vi "VisualizeAnalysis.vi"() -> ()   [LabVIEW 2014, in "Visualization.lvlib" / "VisualizeAnalysis.lvclass"]
uses:
  VisualizeAnalysis.lvclass
  VisualizeBase/VisualizeBase_class/Requests/clUserEventType.ctl
  <vilib>/event_ctls.llb/usereventprio.ctl
  <vilib>/Utility/file.llb/Read From Spreadsheet File (DBL).vi
  <vilib>/Utility/error.llb/Error Cluster From Error Code.vi
  <vilib>/ErrorRing/Error Ring.xnode
  VisualizeBase/VisualizeBase_class/VisualizeBase.lvclass
  <userlib>/NIST/NISTErrorLib/NISTErrorLib.lvlib
  Analysis/AnalysisModule/AnalysisModule.lvlib
panel:
  in  "Pause":bool
  out "Data from file":dbl[][](array[numeric])
  in  "btnOpen":bool
  out "RFE":dbl(graph)
  out "FE":dbl(graph)
  out "Data real time":dbl[](array[numeric])
  out "TVE":dbl[][](graph)
  in  "QueName":string="AnalVisQue"
  out "ErrorArray":errorcluster[](array[cluster])
  in  "btnStop":bool
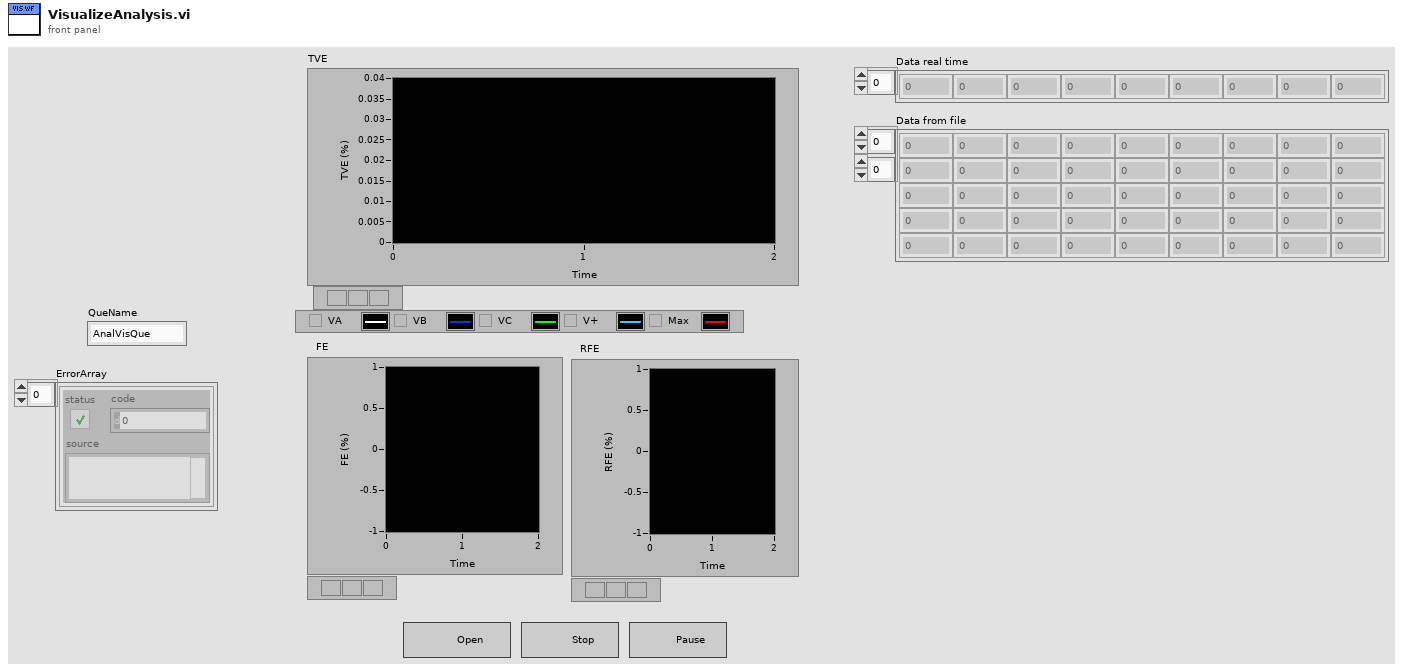
[diagram p1: front panel]
types:
  T1 = typedef "Visualization.lvlib/VisualizeBase.lvclass/clRequestEvents.ctl" = cluster{"StopRequest":refnum<user-event>, "ResetRequest":refnum<user-event>}
  T2 = typedef "AnalysisModule.lvlib/clBroadcastEvents.ctl" = cluster{"DidInit":refnum<user-event>, "StatusUpdate":refnum<user-event>, "ErrorReport":refnum<user-event>, "DidStop":refnum<user-event>, "PathToINI":refnum<user-event>, "Config":refnum<user-event>, "ResultReport":refnum<user-event>}
  T3 = typedef "Visualization.lvlib/VisualizeBase.lvclass/clUserEventType.ctl" = cluster{"BusIndex":i8, "Data":variant}
  T4 = typedef "usereventprio.ctl" = enum32{"high priority", "normal priority"}
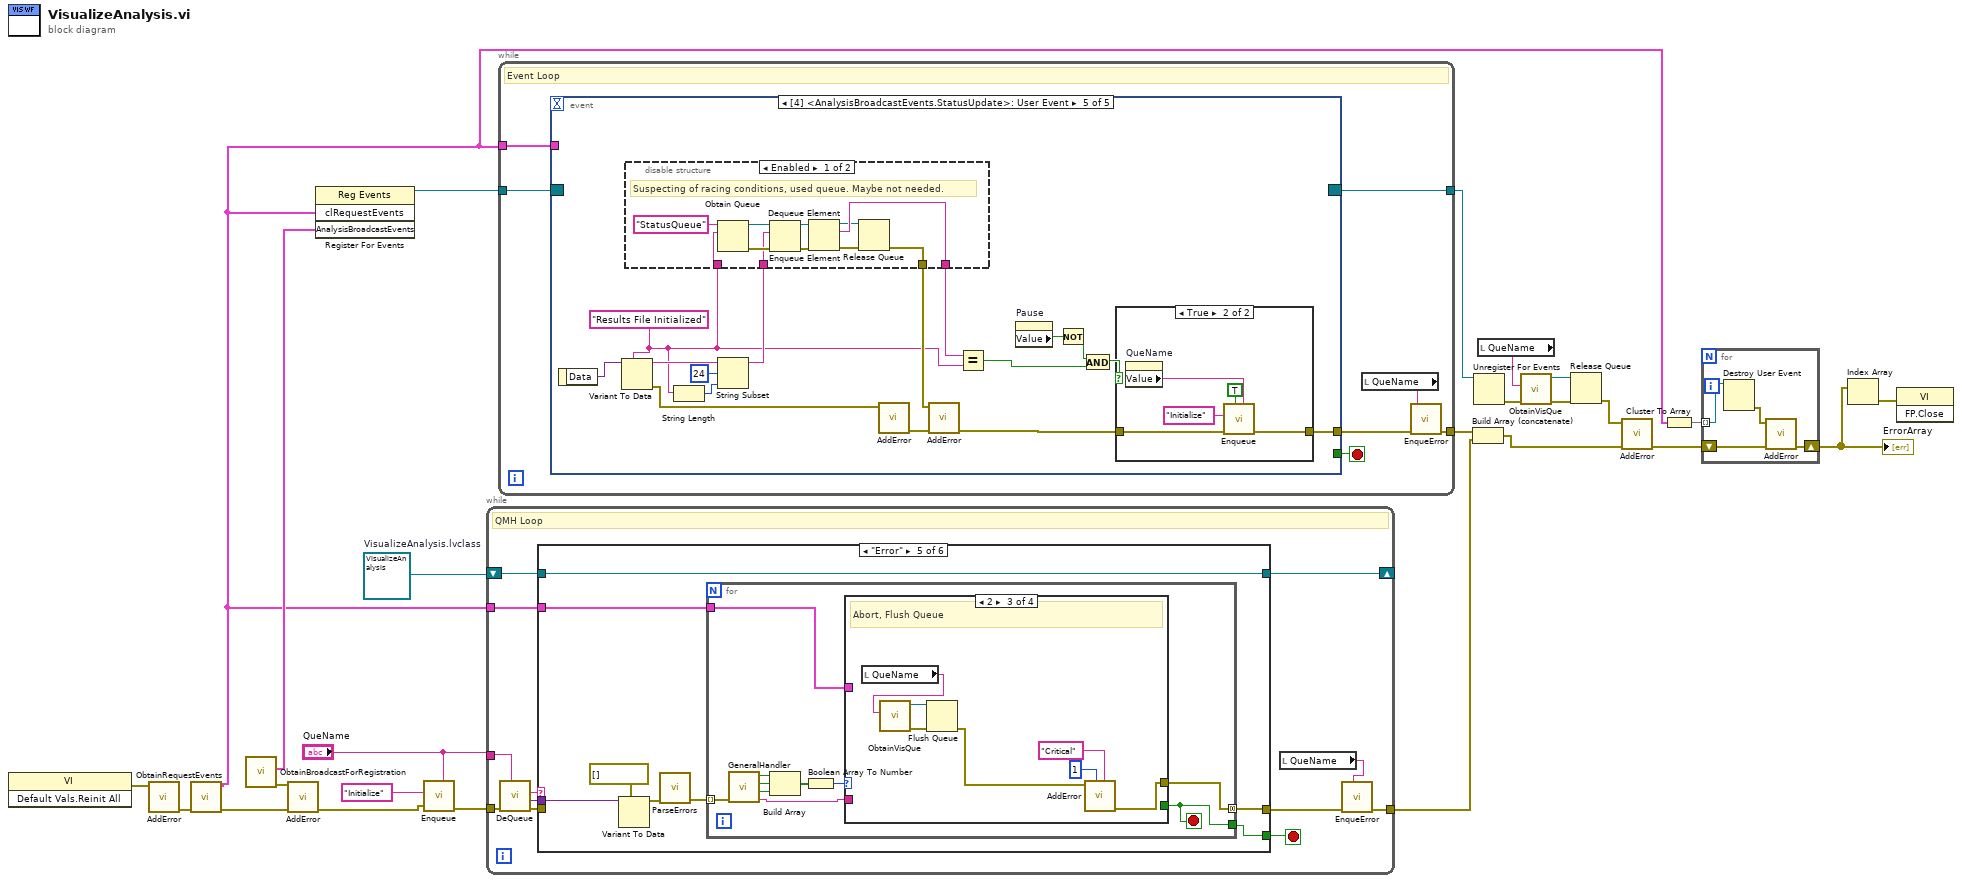
[diagram p0: block diagram]
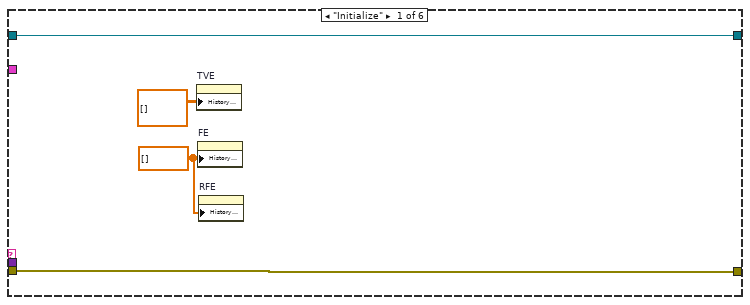
[diagram p2: hidden frame]
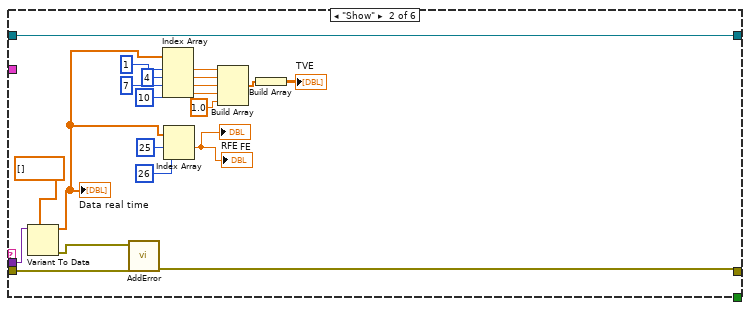
[diagram p3: hidden frame]
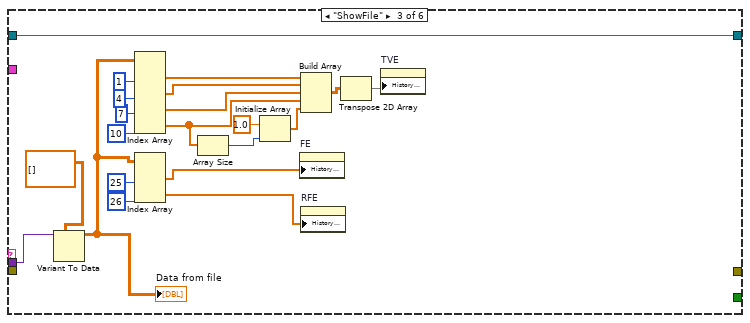
[diagram p4: hidden frame]
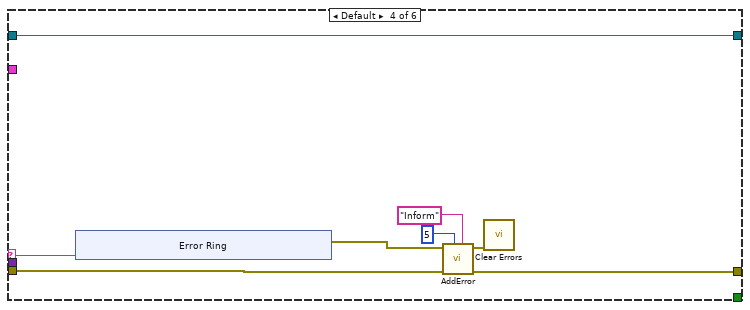
[diagram p5: hidden frame]
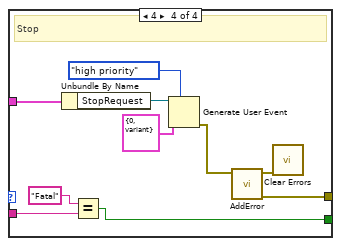
[diagram p8: hidden frame]
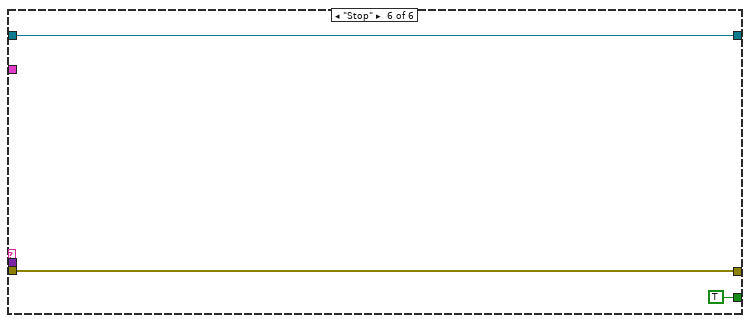
[diagram p9: hidden frame]
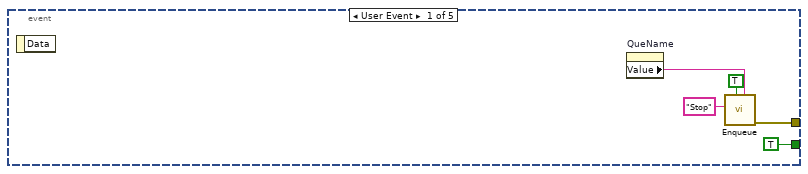
[diagram p10: hidden frame]
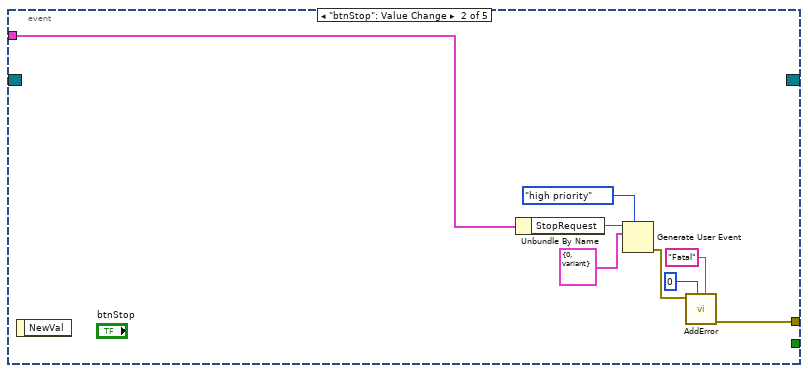
[diagram p11: hidden frame]
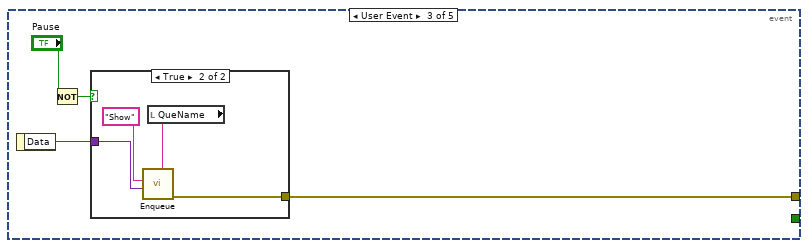
[diagram p12: hidden frame]
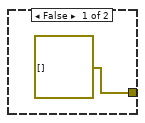
[diagram p13: hidden frame]
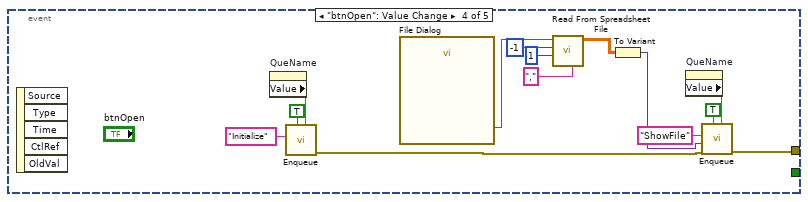
[diagram p14: hidden frame]
diagram:
  w14 = refnum<class "VisualizeAnalysis.lvclass"> refnum  # VisualizeAnalysis.lvclass
  n1 = invoke class="VI" method="Default Vals.Reinit All"() -> (error out=w21:errorcluster)  [unwired: 3 in, 2 out]
  n2 = call <userlib>:"AddError.vi"("error in (no error)"=w21) -> ("ErrorArray"=w20:errorcluster[])  [unwired: 9 in, 1 out]
  n3 = call "ObtainRequestEvents.vi"("Error"=w20) -> ("Error"=w18:errorcluster[], "clRequestEvents"=w1:T1)  [unwired: 9 in]
  n4 = call "ObtainBroadcastForRegistration.vi"() -> ("error out"=w16:errorcluster, "AnalysisBroadcastEvents"=w19:T2)  [unwired: 10 in]
  n5 = call <userlib>:"AddError.vi"("ErrorArray"=w18, "error in (no error)"=w16) -> ("ErrorArray"=w17:errorcluster[])  [unwired: 8 in, 1 out]
  n6 = register-events(w1, w19) -> (reference out=w13:refnum<event-registration>)  [unwired: 2 in, 1 out]
  n7 = call "Enqueue.vi"("QueName"="QueName", "Error"=w17, "Message"="Initialize") -> ("Error"=w24:errorcluster[])  [unwired: 8 in]
  n8 = while {
    tunnel: w24 -> [w37]
    tunnel: [w31] -> w23
    tunnel: "QueName" -> [w29]
    shift-right: [w28] -> _
    shift-left: w14 -> [w27]
    tunnel: w1 -> [w26]
    stop <- w32 stop-if-true
    # "QMH Loop"
    n9 = call "DeQueue.vi"("QueName"=w29, "Error"=w37) -> ("Error"=w34:errorcluster[], "Data"=w35:variant, "Message"=w36:string)  [unwired: 7 in]
    n10 = case shown="\"Error\"" w36 {
      selector: w36 -> [_ _ _ w91 _ _]
      tunnel: w35 -> [_ w61 w83 _ w106 _]
      tunnel: w34 -> [w41 w44 _ w89 _ w135]
      tunnel: [w41 w42 _ w88 w102 w135] -> w33
      tunnel: [_ _ _ _ w101 TRUE] -> w32
      tunnel: w27 -> [w40 w62 w81 w84 w100 w134]
      tunnel: [w40 w62 w81 w84 w100 w134] -> w28
      tunnel: w26 -> [_ _ _ _ w99 _]
      frame "Initialize" {
        w38 = dbl[] [] ("History Data")
        n11 = property on="TVE" class="WFChart (strict)"("History Data"=dbl[][] []) -> ()  [unwired: 2 in, 2 out]
        n12 = property on="FE" class="WFChart (strict)"("History Data"=w38) -> ()  [unwired: 2 in, 2 out]
        n13 = property on="RFE" class="WFChart (strict)"("History Data"=w38) -> ()  [unwired: 2 in, 2 out]
      }
      frame "Show" {
        n14 = Variant To Data(type=dbl[] [], Variant=w61) -> (data=w49:dbl[], error out=w43:errorcluster)  [unwired: 1 in]
        "Data real time" <- w49
        n15 = call <userlib>:"AddError.vi"("ErrorArray"=w44, "error in (no error)"=w43) -> ("ErrorArray"=w42:errorcluster[])  [unwired: 8 in, 1 out]
        n16 = Index Array(array=w49, index #1=1 ("index"), index #2=4 ("index"), index #3=7 ("index"), index #4=10 ("index")) -> (element #1=w58:dbl, element #2=w53:dbl, element #3=w52:dbl, element #4=w45:dbl)
        n17 = Index Array(array=w49, index #1=25 ("index"), index #2=26 ("index")) -> (element #1=→"FE" →"RFE":dbl)  [unwired: 1 out]
        n18 = Build Array(w58, w53, w52, w45, 1.0 ("element")) -> (w57:dbl[])
        n19 = Build Array(w57) -> (→"TVE":dbl[][])
      }
      frame "ShowFile" {
        n20 = Variant To Data(type=dbl[][] [], Variant=w83) -> (data=w71:dbl[][])  [unwired: 1 in, 1 out]
        "Data from file" <- w71
        n21 = Index Array(array=w71, index (col) #1=1 ("disabled index (col)"), index (col) #2=4 ("index (col)"), index (col) #3=7 ("index (col)"), index (col) #4=10 ("index (col)")) -> (element #1=w76:dbl[], element #2=w75:dbl[], element #3=w74:dbl[], element #4=w66:dbl[])  [unwired: 4 in]
        n22 = Index Array(array=w71, index (col) #1=25 ("disabled index (col)"), index (col) #2=26 ("index (col)")) -> (element #1=w68:dbl[], element #2=w67:dbl[])  [unwired: 2 in]
        n23 = Array Size(array=w66) -> (size(s)=w65:i32)
        n24 = Initialize Array(1.0 ("element"), w65) -> (w63:dbl[])
        n25 = property on="FE" class="WFChart (strict)"("History Data"=w68) -> ()  [unwired: 2 in, 2 out]
        n26 = Build Array(w76, w75, w74, w66, w63) -> (w73:dbl[][])
        n27 = property on="RFE" class="WFChart (strict)"("History Data"=w67) -> ()  [unwired: 2 in, 2 out]
        n28 = Transpose 2D Array(2D array=w73) -> (transposed array=w72:dbl[][])
        n29 = property on="TVE" class="WFChart (strict)"("History Data"=w72) -> ()  [unwired: 2 in, 2 out]
      }
      frame Default {
        n30 = xnode "Error Ring"("parameter 0"=w91) -> ("error out"=w90:errorcluster)
        n31 = call <userlib>:"AddError.vi"("Severity"="Inform" ("String"), "Priority"=u8 5, "ErrorArray"=w89, "error in (no error)"=w90) -> ("ErrorArray"=w88:errorcluster[], "error out"=w87:errorcluster)  [unwired: 6 in]
        n32 = call <vilib>:"Clear Errors.vi"("error in (no error)"=w87) -> ()  [unwired: 5 in, 2 out]
      }
      frame "Error" {
        n33 = Variant To Data(type=errorcluster[] [], Variant=w106) -> (data=w104:errorcluster[])  [unwired: 1 in, 1 out]
        n34 = call <userlib>:"ParseErrors.vi"("ErrorArray"=w104) -> ("ErrorArray"=w103:errorcluster[])  [unwired: 8 in, 2 out]
        n35 = for {
          tunnel: w103 -> [w116] mode=indexing
          tunnel: [w110] -> w102 mode=concatenating
          tunnel: [w108] -> w101
          tunnel: w99 -> [w107]
          stop <- w108 stop-if-true
          n36 = call <userlib>:"GeneralHandler.vi"("error in (no error)"=w116) -> ("Severity"=w109:string, "Stop"=w113:bool, "Abort"=w114:bool, "Continue"=w115:bool)  [unwired: 7 in]
          n37 = Build Array(w115, w114, w113) -> (w112:bool[])
          n38 = Boolean Array To Number(Boolean array=w112) -> (number=w111:u32)
          n39 = case shown="2" w111 {
            tunnel: [_ _ w121 w132] -> w110
            tunnel: w109 -> [_ _ _ w127]
            tunnel: [_ _ _ w125] -> w108
            tunnel: w107 -> [_ _ _ w124]
            frame 0, Default {
              # "No Dialog"
            }
            frame 1 {
              # "Continue"
            }
            frame 2 {
              # "Abort, Flush Queue"
              n40 = local read "QueName"() -> (w117:string)
              n41 = call "ObtainVisQue.vi"("QueName"=w117) -> ("error out"=w123:errorcluster, "queue out"=w122:refnum<queue>)  [unwired: 9 in]
              n42 = Flush Queue(queue=w122, error in (no error)=w123) -> (error out=w120:errorcluster)  [unwired: 2 out]
              n43 = call <userlib>:"AddError.vi"("Severity"="Critical" ("String"), "Priority"=u8 1, "error in (no error)"=w120) -> ("ErrorArray"=w121:errorcluster[])  [unwired: 7 in, 1 out]
            }
            frame 4 {
              # "Stop"
              n44 = Unbundle By Name(w124) -> ("StopRequest"=w133:refnum<user-event>)
              n45 = Equal?(x="Fatal", y=w127) -> (x = y?=w125:bool)
              n46 = Generate User Event(priority (normal)=usereventprio."high priority", user event=w133, event data cluster=T3 {"BusIndex"=0, "Data"=variant} ("event data")) -> (error out=w131:errorcluster)  [unwired: 1 in, 1 out]
              n47 = call <userlib>:"AddError.vi"("error in (no error)"=w131) -> ("ErrorArray"=w132:errorcluster[], "error out"=w128:errorcluster)  [unwired: 9 in]
              n48 = call <vilib>:"Clear Errors.vi"("error in (no error)"=w128) -> ()  [unwired: 5 in, 2 out]
            }
          }
        }
      }
      frame "Stop" {
      }
    }
    n49 = local read "QueName"() -> (w30:string)
    n50 = call "EnqueError.vi"("QueName"=w30, "Error"=w33) -> ("Error"=w31:errorcluster[])  [unwired: 9 in]
  }
  n51 = while {
    tunnel: [w141] -> w22
    tunnel: w13 -> [w139]
    tunnel: [w138] -> w7
    tunnel: w1 -> [w137]
    stop <- w143 stop-if-true
    # "Event Loop"
    n52 = event shown="[4] <AnalysisBroadcastEvents.StatusUpdate>: User Event" {
      selector: w139 -> [_ _ _ _ _]
      dyn-events: [_ _ _ _ _] -> w138
      timeout: _ -> [_ _ _ _ _]
      tunnel: [TRUE _ _ _ _] -> w143
      tunnel: [w147 w154 w159 w174 w194] -> w142
      tunnel: w137 -> [_ w149 _ _ _]
      event User Event {
        n53 = event-data() -> ()  [unwired: 1 in, 1 out]
        n54 = property on="QueName" class="Str"() -> ("Value"=w144:string)  [unwired: 2 in, 2 out]
        n55 = call "Enqueue.vi"("QueName"=w144, "Priority? (F)"=TRUE, "Message"="Stop") -> ("Error"=w147:errorcluster[])  [unwired: 8 in]
      }
      event "btnStop": Value Change {
        n56 = event-data() -> ()  [unwired: 1 in, 1 out]
        n57 = Unbundle By Name(w149) -> ("StopRequest"=w155:refnum<user-event>)
        n58 = Generate User Event(priority (normal)=usereventprio."high priority", user event=w155, event data cluster=T3 {"BusIndex"=0, "Data"=variant} ("event data")) -> (error out=w156:errorcluster)  [unwired: 1 in, 1 out]
        n59 = call <userlib>:"AddError.vi"("Severity"="Fatal" ("String"), "Priority"=u8 0, "error in (no error)"=w156) -> ("ErrorArray"=w154:errorcluster[])  [unwired: 7 in, 1 out]
      }
      event User Event {
        n60 = event-data() -> ("Data"=w160:variant)  [unwired: 1 in]
        n61 = Not(x="Pause") -> (.not. x?=w157:bool)
        n62 = case shown="True" w157 {
          tunnel: w160 -> [_ w164]
          tunnel: [errorcluster[] [] ("Error") w163] -> w159
          frame False {
          }
          frame True {
            n63 = local read "QueName"() -> (w165:string)
            n64 = call "Enqueue.vi"("QueName"=w165, "Data"=w164, "Message"="Show") -> ("Error"=w163:errorcluster[])  [unwired: 8 in]
          }
        }
      }
      event "btnOpen": Value Change {
        n65 = event-data() -> ()  [unwired: 1 in, 5 out]
        n66 = property on="QueName" class="Str"() -> ("Value"=w171:string)  [unwired: 2 in, 2 out]
        n67 = call "Enqueue.vi"("QueName"=w171, "Priority? (F)"=TRUE, "Message"="Initialize") -> ("Error"=w168:errorcluster[])  [unwired: 8 in]
        n68 = call "File Dialog"() -> ("selected path"=w179:path)  [unwired: 12 in, 3 out]
        n69 = call-poly <vilib>:"Read From Spreadsheet File.vi"("delimiter (\\t)"="," ("delimiter (\\t)"), "start of read offset (chars.:0)"=1, "number of rows (all:-1)"=-1, "file path (dialog if empty)"=w179) -> ("all rows"=w173:dbl[][])  [unwired: 3 in, 4 out]
        n70 = To Variant(anything=w173) -> (Variant=w172:variant)
        n71 = property on="QueName" class="Str"() -> ("Value"=w175:string)  [unwired: 2 in, 2 out]
        n72 = call "Enqueue.vi"("QueName"=w175, "Priority? (F)"=TRUE, "Error"=w168, "Data"=w172, "Message"="ShowFile") -> ("Error"=w174:errorcluster[])  [unwired: 6 in]
      }
      event User Event {
        w184 = "Results File Initialized" ("Status")
        n73 = event-data() -> ("Data"=w195:variant)  [unwired: 1 in]
        n74 = Variant To Data(type=w184, Variant=w195) -> (data=w192:string, error out=w189:errorcluster)  [unwired: 1 in]
        n75 = String Length(string=w184) -> (length=w185:i32)
        n76 = String Subset(string=w192, offset (0)=24, length (rest)=w185) -> (substring=w187:string)
        n77 = disable-structure shown="Enabled" {
          disable-tunnel: [w199 w207] -> w191
          disable-tunnel: [w196 _] -> w188
          disable-tunnel: w187 -> [w201 w207]
          disable-tunnel: w184 -> [w200 _]
          frame Enabled {
            # "Suspecting of racing conditions, used queue. Maybe not needed."
            n78 = Obtain Queue(name (unnamed)="StatusQueue", element data type=w200) -> (queue out=w205:refnum<queue>, error out=w203:errorcluster)  [unwired: 3 in, 1 out]
            n79 = Enqueue Element(queue=w205, element=w201, error in (no error)=w203) -> (queue out=w204:refnum<queue>, error out=w202:errorcluster)  [unwired: 1 in, 1 out]
            n80 = Dequeue Element(queue=w204, error in (no error)=w202) -> (queue out=w198:refnum<queue>, element=w199:string, error out=w197:errorcluster)  [unwired: 1 in, 1 out]
            n81 = Release Queue(queue=w198, error in (no error)=w197) -> (error out=w196:errorcluster)  [unwired: 1 in, 2 out]
          }
          frame Disabled {
          }
        }
        n82 = call <userlib>:"AddError.vi"("error in (no error)"=w189) -> ("ErrorArray"=w190:errorcluster[])  [unwired: 9 in, 1 out]
        n83 = call <userlib>:"AddError.vi"("ErrorArray"=w190, "error in (no error)"=w188) -> ("ErrorArray"=w193:errorcluster[])  [unwired: 8 in, 1 out]
        n84 = Equal?(x=w191, y=w184) -> (x = y?=w182:bool)
        n85 = property on="Pause" class="Bool (strict)"() -> ("Value"=w181:bool)  [unwired: 2 in, 2 out]
        n86 = Not(x=w181) -> (.not. x?=w180:bool)
        n87 = And(x=w180, y=w182) -> (x .and. y?=w183:bool)
        n88 = case shown="True" w183 {
          tunnel: [w208 w210] -> w194
          tunnel: w193 -> [w208 w209]
          frame False {
          }
          frame True {
            n89 = property on="QueName" class="Str"() -> ("Value"=w211:string)  [unwired: 2 in, 2 out]
            n90 = call "Enqueue.vi"("QueName"=w211, "Priority? (F)"=TRUE, "Error"=w209, "Message"="Initialize") -> ("Error"=w210:errorcluster[])  [unwired: 7 in]
          }
        }
      }
    }
    n91 = local read "QueName"() -> (w140:string)
    n92 = call "EnqueError.vi"("QueName"=w140, "Error"=w142) -> ("Error"=w141:errorcluster[])  [unwired: 9 in]
  }
  n93 = Build Array (concatenate)(w22, w23) -> (w6:errorcluster[])
  n94 = Unregister For Events(event registration refnum=w7) -> (error out=w9:errorcluster)  [unwired: 1 in]
  n95 = local read "QueName"() -> (w3:string)
  n96 = call "ObtainVisQue.vi"("error in (no error)"=w9, "QueName"=w3) -> ("error out"=w10:errorcluster, "queue out"=w11:refnum<queue>)  [unwired: 8 in]
  n97 = Release Queue(queue=w11, error in (no error)=w10) -> (error out=w12:errorcluster)  [unwired: 1 in, 2 out]
  n98 = call <userlib>:"AddError.vi"("ErrorArray"=w6, "error in (no error)"=w12) -> ("ErrorArray"=w2:errorcluster[])  [unwired: 8 in, 1 out]
  n99 = Cluster To Array(cluster=w1) -> (array=w8:refnum<user-event>[])
  n100 = for {
    tunnel: w8 -> [w217] mode=indexing
    shift-right: [w216] -> w5
    shift-left: w2 -> [w215]
    n101 = Destroy User Event(user event=w217) -> (error out=w214:errorcluster)  [unwired: 1 in]
    n102 = call <userlib>:"AddError.vi"("ErrorArray"=w215, "error in (no error)"=w214) -> ("ErrorArray"=w216:errorcluster[])  [unwired: 8 in, 1 out]
  }
  "ErrorArray" <- w5
  n103 = Index Array(array=w5) -> (element=w4:errorcluster)  [unwired: 1 in]
  n104 = invoke class="VI" method="FP.Close"(error in=w4) -> ()  [unwired: 2 in, 3 out]
